vi "readPruebasFromCSV.vi"(5 "Equipos":string(combo), 11 "error in (no error)":errorcluster) -> (4 "Prueba out":refnum<class "Prueba.lvclass">, 10 "Descripcion":string[](array[string]), 15 "error out":errorcluster)   [LabVIEW 2019, in "Prueba.lvclass"]
uses:
  Prueba.lvclass
  <vilib>/Utility/file.llb/Read Delimited Spreadsheet (string).vi
panel:
  out "Prueba":string[](array[string])
  out "all rows":string[][](array[string])
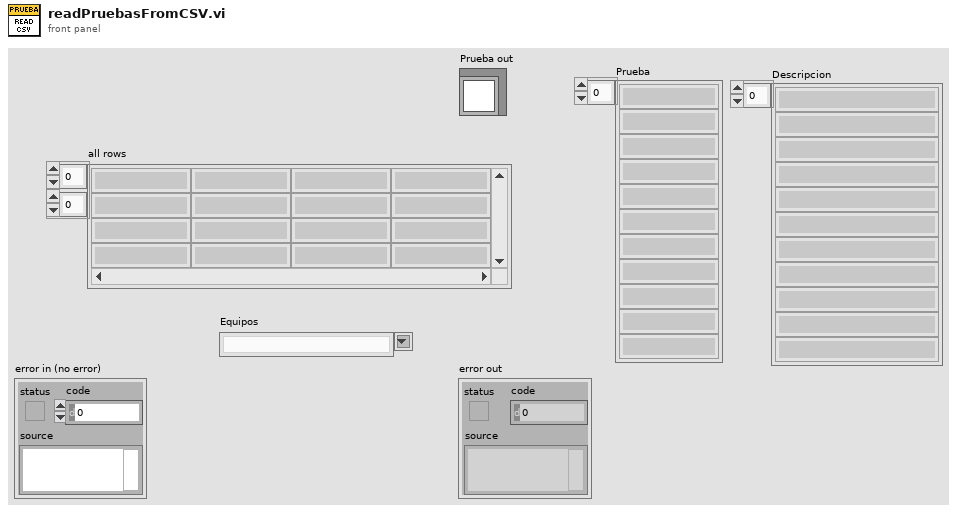
[diagram p1: front panel]
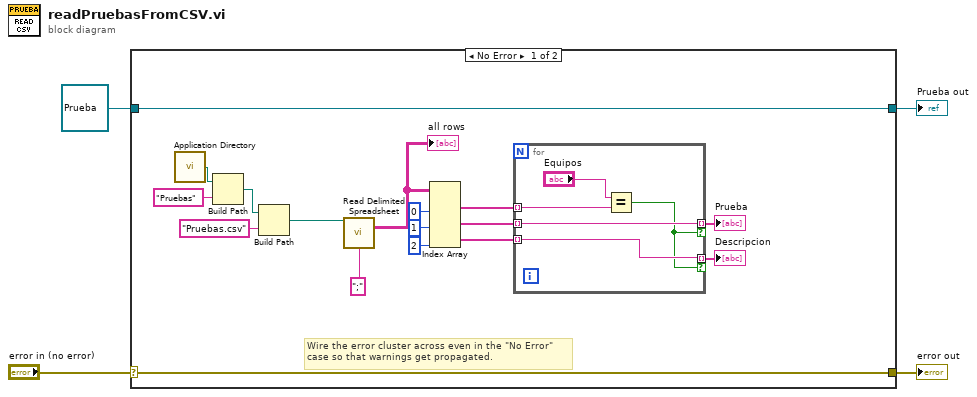
[diagram p0: block diagram]
diagram:
  n1 = case shown="No Error" "error in (no error)" {
    selector: "error in (no error)" -> [w20 w28]
    tunnel: [w20 w28] -> w3
    tunnel: [w21 w27] -> w1
    tunnel: refnum<class "Prueba.lvclass"> refnum ("Prueba in") -> [w21 w27]
    frame No Error {
      # "Wire the error cluster across even in the \"No Error\"\ncase so that warnings get propagated."
      n2 = call <vilib>:"Application Directory.vi"() -> ("Application Directory"=w19:path)
      n3 = Build Path(base path=w19, name or relative path="Pruebas") -> (appended path=w17:path)
      n4 = Build Path(base path=w17, name or relative path="Pruebas.csv") -> (appended path=w15:path)
      n5 = call-poly <vilib>:"Read Delimited Spreadsheet.vi"("file path (dialog if empty)"=w15, "delimiter (\\t)"=";" ("delimiter (\\t)")) -> ("all rows"=w13:string[][])  [unwired: 8 in, 5 out]
      "all rows" <- w13
      n6 = Index Array(array=w13, index (col) #1=0 ("disabled index (col)"), index (col) #2=1 ("index (col)"), index (col) #3=2 ("index (col)")) -> (element #1=w9:string[], element #2=w8:string[], element #3=w7:string[])  [unwired: 3 in]
      n7 = for {
        tunnel: w9 -> [w25] mode=indexing
        tunnel: w8 -> [w24] mode=indexing
        tunnel: w7 -> [w23] mode=indexing
        tunnel: [w24] -> w6 mode=indexing if=w22
        tunnel: [w23] -> w5 mode=indexing if=w22
        n8 = Equal?(x="Equipos", y=w25) -> (x = y?=w22:bool)
      }
      "Prueba" <- w6
      "Descripcion" <- w5
    }
    frame Error {
    }
  }
  "error out" <- w3
  "Prueba out" <- w1
